vi "Runtime Testing.vi"() -> ()   [LabVIEW 2013, in "tag select module tests.lvlib"]
uses:
  tag select module tests.lvlib
  module/execution/tag select module runtime.lvclass
  module/execution/tag select module runtime.lvclass/tag select module runtime.ctl
  <vilib>/NI/Tag Bus/table/data polymorphs/write one/write Boolean.vi
  <vilib>/NI/Tag Bus/table/data polymorphs/write one/write Double.vi
  <vilib>/NI/Tag Bus/table/data polymorphs/read one/read Double.vi
  module/execution/Read tag select.vi
  <vilib>/NI/Tag Bus/table/data table.lvlib
panel:
  out "out":dbl
  in  "result":bool
  in  "Select":bool
  in  "b":dbl
  in  "a":dbl
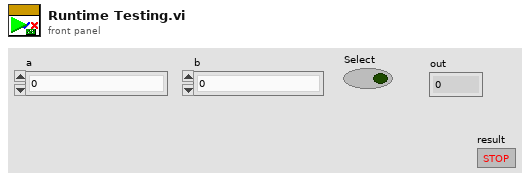
[diagram p1: front panel]
types:
  T1 = typedef "TBM channel.lvclass/data tables.ctl" = cluster{"input data":T2, "processing parameter":T2, "processing result":T2, "output data":T2}
  T2 = typedef "tag bus.lvlib/dictionary table pair.ctl" = cluster{"data dictionary":refnum<class "data dictionary.lvclass">, "data table":T3}
  T3 = typedef "tag bus.lvlib/data table.lvlib/data table.ctl" = cluster{"Double":dbl[], "Single":sgl[], "I64":i64[], "I32":i32[], "I16":i16[], "I8":i8[], "U64":u64[], "U32":u32[], "U16":u16[], "U8":u8[], "Boolean":bool[], "String":string[], "Array of Double":cluster{"DBL Array":dbl[]}[], "Array of Single":cluster{"SGL Array":sgl[]}[], "Array of I64":cluster{"I64 Array":i64[]}[], "Array of I32":cluster{"I32 Array":i32[]}[], "Array of I16":cluster{"I16 Array":i16[]}[], "Array of I8":cluster{"I8 Array":i8[]}[], "Array of U64":cluster{"U64 Array":u64[]}[], "Array of U32":cluster{"U32 Array":u32[]}[], "Array of U16":cluster{"U16 Array":u16[]}[], "Array of U8":cluster{"U8 Array":u8[]}[], "Array of Boolean":cluster{"Boolean Array":bool[]}[], "Array of String":cluster{"String Array":string[]}[]}
  T4 = typedef "runtime tag select configuration.ctl" = cluster{"output index":i32, "select index (bool)":i32, "input index":i32[], "data type":T5}
  T5 = typedef "tag bus.lvlib/tag descriptor.lvclass/Data Type.ctl" = enum16{"Double", "Single", "I64", "I32", "I16", "I8", "U64", "U32", "U16", "U8", "Boolean", "String", "Array of Double", "Array of Single", "Array of I64", "Array of I32", "Array of I16", "Array of I8", "Array of U64", "Array of U32", "Array of U16", "Array of U8", "Array of Boolean", "Array of String"}
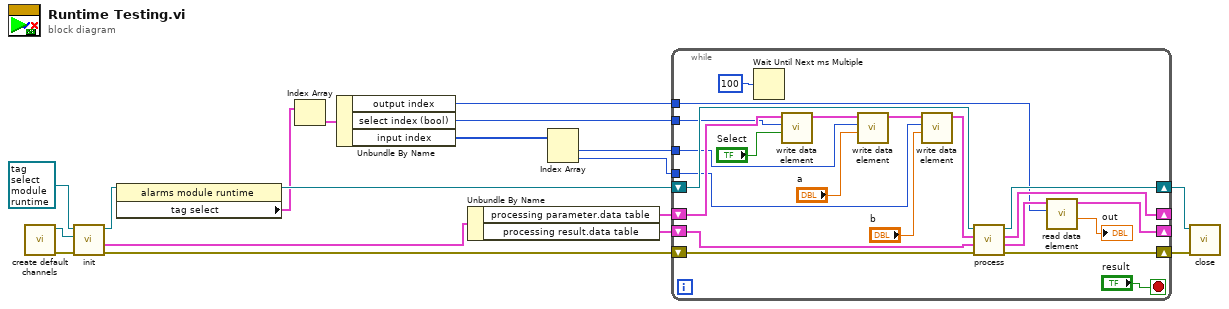
[diagram p0: block diagram]
diagram:
  n1 = call "create default channels.vi"() -> ("error out"=w16:errorcluster, "module"=w18:refnum<class "tag select module configuration.lvclass">)  [unwired: 8 in, 2 out]
  n2 = call-dynamic "init.vi"("error in"=w16, "TBM module configuration in"=w18, "tag select module runtime in"=refnum<class "tag select module runtime.lvclass"> refnum ("tag bus configurable plugin module")) -> ("error out"=w13:errorcluster, "data allocations"=w12:T1, "tag select module runtime out"=w9:refnum<class "tag select module runtime.lvclass">)  [unwired: 5 in, 1 out]
  n3 = property class="alarms module runtime"(reference=w9) -> (reference out=w8:refnum<class "tag select module runtime.lvclass">, "tag select"=w7:T4[])  [unwired: 1 in, 1 out]
  n4 = Index Array(array=w7) -> (element=w6:T4)  [unwired: 1 in]
  n5 = Unbundle By Name(w6) -> ("output index"=w5:i32, "select index (bool)"=w1:i32, "input index"=w2:i32[])
  n6 = Unbundle By Name(w12) -> ("processing parameter.data table"=w11:T3, "processing result.data table"=w10:T3)
  n7 = Index Array(array=w2) -> (element #1=w4:i32, element #2=w3:i32)  [unwired: 2 in]
  n8 = while {
    shift-right: [w39] -> w14
    shift-left: w8 -> [w40]
    shift-right: [w37] -> w15
    shift-left: w13 -> [w38]
    shift-right: [w36] -> _
    shift-left: w11 -> [w32]
    shift-right: [w29] -> _
    shift-left: w10 -> [w35]
    tunnel: w5 -> [w22]
    tunnel: w3 -> [w21]
    tunnel: w4 -> [w20]
    tunnel: w1 -> [w19]
    stop <- "result" stop-if-true
    n9 = Wait Until Next ms Multiple(millisecond multiple=u32 100) -> ()  [unwired: 1 out]
    n10 = call-poly <vilib>:"write data element.vi"("value"="Select", "index"=w19, "data table in"=w32) -> ("data table out"=w33:T3)  [unwired: 8 in]
    n11 = call-poly <vilib>:"write data element.vi"("value"="a", "index"=w20, "data table in"=w33) -> ("data table out"=w34:T3)  [unwired: 8 in]
    n12 = call-poly <vilib>:"write data element.vi"("value"="b", "index"=w21, "data table in"=w34) -> ("data table out"=w31:T3)  [unwired: 8 in]
    n13 = call-dynamic "process.vi"("error in"=w38, "result allocation"=w35, "parameters"=w31, "module in"=w40) -> ("error out"=w37:errorcluster, "results"=w30:T3, "parameter allocation"=w36:T3, "module out"=w39:refnum<class "tag select module runtime.lvclass">)  [unwired: 4 in]
    n14 = call-poly <vilib>:"read data element.vi"("index"=w22, "data table in"=w30) -> ("value"=→"out":dbl, "data table out"=w29:T3)  [unwired: 8 in]
  }
  n15 = call-dynamic "close.vi"("error in"=w15, "alarms module runtime in"=w14) -> ()  [unwired: 9 in, 1 out]
